vi "Log Cryogen (No Objects).vi"(8 "error in (no error)":errorcluster, 10 "Status string":string="Needle Valve", 11 "Cluster In":T3={"helium"={"fastHe?"=FALSE, "slowHe?"=FALSE, "fillHe?"=FALSE, "lowHe?"=FALSE}, "nitrogen"={"fillN?"=FALSE, "lowN?"=FALSE}, "Shutdown"=FALSE, "Cryogen Levels"=[], "IO Info"={"Address"={"Com Port"=1, "ISOBUS Address"=5, "GPIB Address"=24, "Communication"=enum."ISOBUS"}, "ILM Name"="", "Display Channel"=[]}} {"Cryogen Levels" min=-1.0 max=100.0 scale=0.0..100.0}) -> (0 "error out":errorcluster, 3 "Cluster Out":T3={"helium"={"fastHe?"=FALSE, "slowHe?"=FALSE, "fillHe?"=FALSE, "lowHe?"=FALSE}, "nitrogen"={"fillN?"=FALSE, "lowN?"=FALSE}, "Shutdown"=FALSE, "Cryogen Levels"=[], "IO Info"={"Address"={"Com Port"=1, "ISOBUS Address"=5, "GPIB Address"=24, "Communication"=enum."ISOBUS"}, "ILM Name"="", "Display Channel"=[]}} {"Cryogen Levels" min=-1.0 max=100.0 scale=0.0..100.0})   [LabVIEW 2012]
uses:
  Cryogen Levels.ctl
  Oxford/BUSGEN.LLB/OxfordAddress.ctl
  Global/File Locations.vi
  Level Meter.lvclass
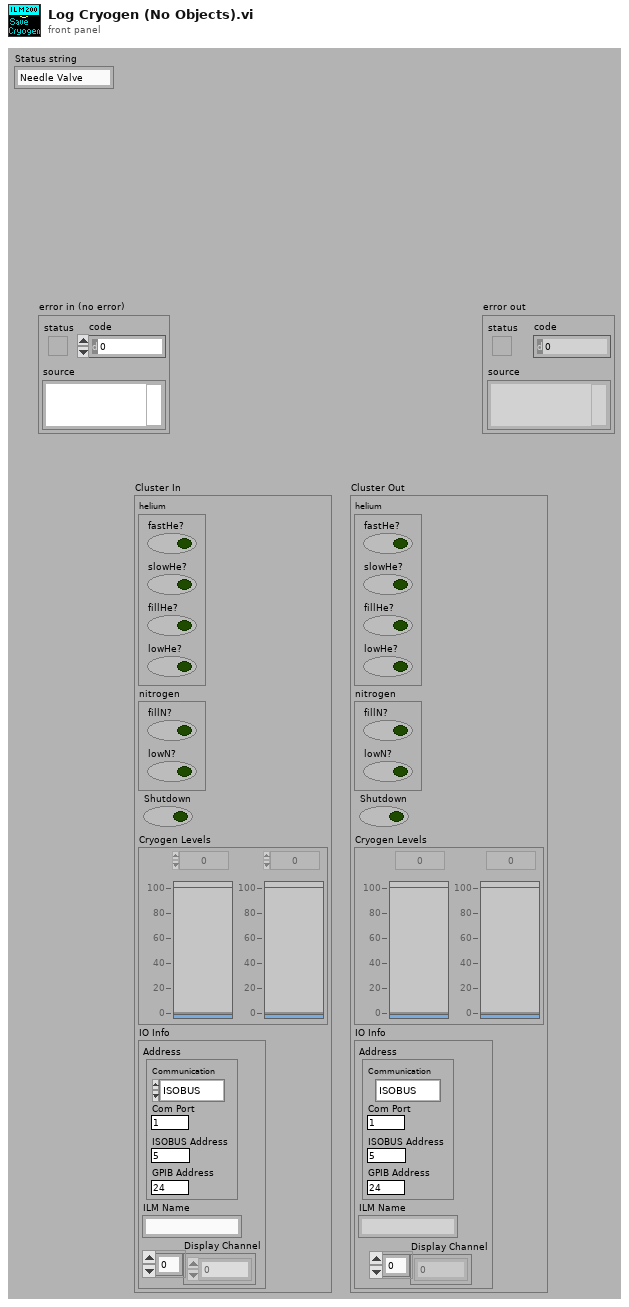
[diagram p1: front panel]
types:
  T1 = typedef "Level Meter.lvclass/Cryogen Levels.ctl" = dbl[]
  T2 = typedef "OxfordAddress.ctl" = cluster{"Com Port":i32, "ISOBUS Address":i32, "GPIB Address":i16, "Communication":enum16{"RS232", "ISOBUS", "GPIB", "Gateway"}}
  T3 = cluster{"helium":cluster{"fastHe?":bool, "slowHe?":bool, "fillHe?":bool, "lowHe?":bool}, "nitrogen":cluster{"fillN?":bool, "lowN?":bool}, "Shutdown":bool, "Cryogen Levels":T1, "IO Info":cluster{"Address":T2, "ILM Name":string, "Display Channel":i32[]}}
  T4 = enum16{"open", "open or create", "create or replace", "create", "open (read only)"}
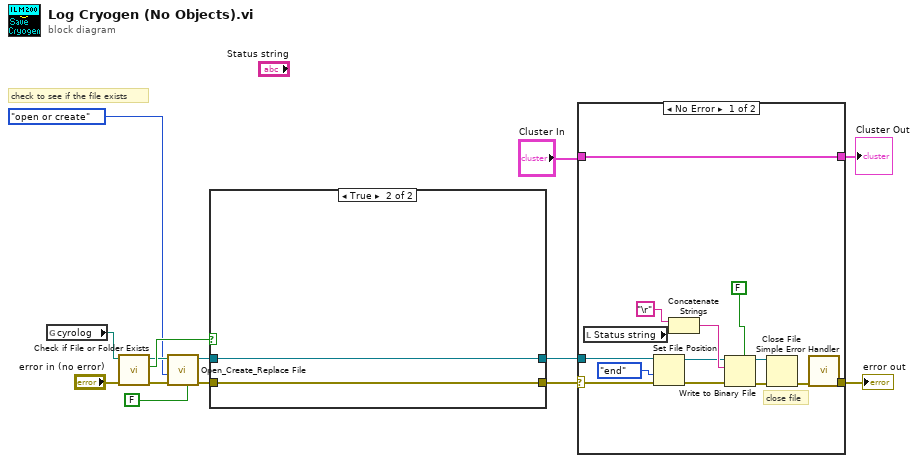
[diagram p0: block diagram]
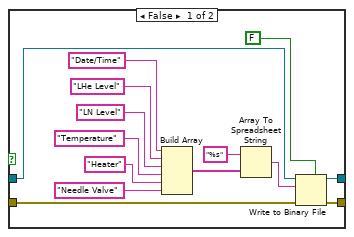
[diagram p3: hidden frame]
diagram:
  # "check to see if the file exists"
  n1 = global read "File Locations.vi" "cyrolog"() -> (w14:path)
  n2 = call <vilib>:"Check if File or Folder Exists.vi"("error in (no error)"="error in (no error)", "path"=w14) -> ("error out"=w6:errorcluster, "file or folder exists?"=w10:bool, "dup path"=w9:path)  [unwired: 7 out]
  n3 = call <vilib>:"Open_Create_Replace File.vi"("advisory dialog? (display:T)"=FALSE, "error in (no error)"=w6, "function (open:0)"=T4."open or create", "file path"=w9) -> ("error out"=w7:errorcluster, "refnum"=w8:refnum<file>)  [unwired: 3 in, 3 out]
  n4 = case shown="True" w10 {
    tunnel: w8 -> [w28 w30]
    tunnel: w7 -> [w27 w29]
    tunnel: [w20 w30] -> w13
    tunnel: [w19 w29] -> w12
    frame False {
      n5 = Build Array("Date/Time", "LHe Level", "LN Level", "Temperature", "Heater", "Needle Valve") -> (w16:string[])
      n6 = Array To Spreadsheet String(array=w16, 3:"%s" ("format string")) -> (spreadsheet string=w15:string)  [unwired: 1 in]
      n7 = Write to Binary File(file (use dialog)=w28, data=w15, error in=w27, 5:FALSE ("prepend array or string size? (T)")) -> (refnum out=w20:refnum<file>, error out=w19:errorcluster)  [unwired: 3 out]
    }
    frame True {
    }
  }
  n8 = case shown="No Error" w12 {
    selector: w12 -> [w37 w45]
    tunnel: w13 -> [w43 _]
    tunnel: "Cluster In" -> [w38 w46]
    tunnel: [w38 w46] -> w1
    tunnel: [w39 w45] -> w3
    frame No Error {
      # "close file"
      n9 = local read "Status string"() -> (w34:string)
      n10 = Set File Position(refnum=w43, from (0:start)=enum16{"start", "end", "current"}."end", error in=w37) -> (refnum out=w32:refnum<file>, error out=w31:errorcluster)  [unwired: 1 out]
      n11 = Concatenate Strings("\r", w34) -> (w33:string)
      n12 = Write to Binary File(file (use dialog)=w32, data=w33, error in=w31, 5:FALSE ("prepend array or string size? (T)")) -> (refnum out=w44:refnum<file>, error out=w42:errorcluster)  [unwired: 3 out]
      n13 = Close File(refnum=w44, error in=w42) -> (error out=w41:errorcluster)  [unwired: 1 out]
      n14 = call <vilib>:"Simple Error Handler.vi"("error in (no error)"=w41) -> ("error out"=w39:errorcluster)  [unwired: 4 in, 4 out]
    }
    frame Error {
    }
  }
  "error out" <- w3
  "Cluster Out" <- w1
